vi "Start.vi"(8 "error in (no error)":errorcluster, 11 "Virt Instr Base in":refnum<class "Virt Instr Base.lvclass">) -> (0 "error out":errorcluster, 3 "Virt Instr Base out":refnum<class "Virt Instr Base.lvclass">)   [LabVIEW 2023, in "HAL GOOP4.lvlib" / "Virt Instr Base.lvclass"]
uses:
  Virt Instr Base.lvclass
  Virt Instr Base.lvclass/Virt Instr Base.ctl
  Instrument/Instrument.lvclass
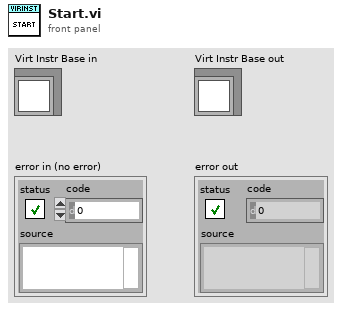
[diagram p1: front panel]
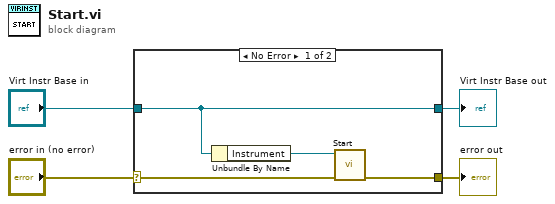
[diagram p0: block diagram]
diagram:
  n1 = case shown="No Error" "error in (no error)" {
    selector: "error in (no error)" -> [w7 w10]
    tunnel: [w6 w10] -> w3
    tunnel: [w5 w9] -> w1
    tunnel: "Virt Instr Base in" -> [w5 w9]
    frame No Error {
      n2 = Unbundle By Name(w5) -> ("Instrument"=w8:refnum<class "Instrument.lvclass">)
      n3 = call "Start.vi"("error in (no error)"=w7, "reference in"=w8) -> ("error out"=w6:errorcluster)  [unwired: 8 in, 1 out]
    }
    frame Error {
    }
  }
  "error out" <- w3
  "Virt Instr Base out" <- w1
